vi "Write TCPClient.vi"(8 "error in (no error)":errorcluster, 10 "TCPClient.lvclass":refnum<class "TCPClient.lvclass">, 11 "MonoClient in":refnum<class "MonoClientCommunicator.lvclass">) -> (0 "error out":errorcluster, 3 "MonoClient out":refnum<class "MonoClientCommunicator.lvclass">)   [LabVIEW 2016, in "MonoClientCommunicator.lvclass"]
uses:
  MonoClientCommunicator.lvclass
  ts_labview_tcp/TCPClient/TCPClient.lvclass
  MonoClientCommunicator.lvclass/MonoClientCommunicator.ctl
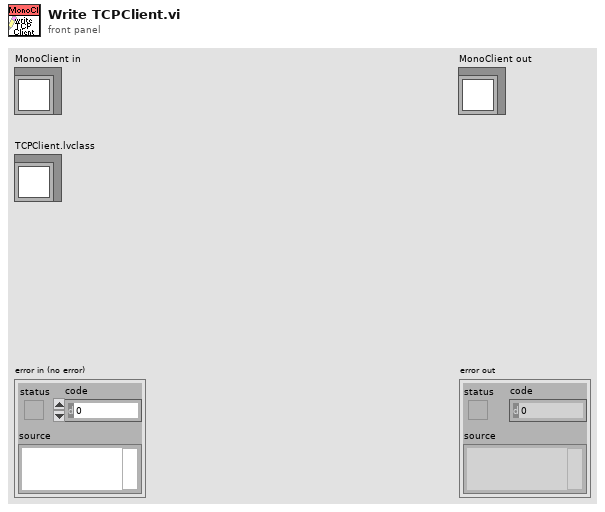
[diagram p1: front panel]
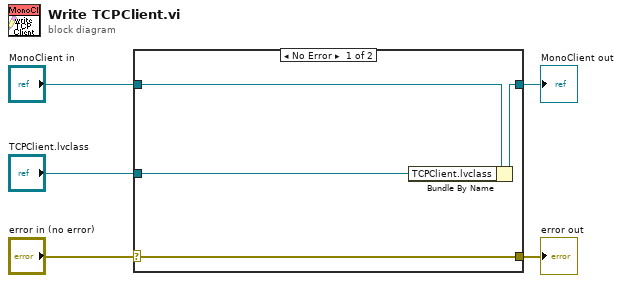
[diagram p0: block diagram]
diagram:
  n1 = case shown="No Error" "error in (no error)" {
    selector: "error in (no error)" -> [w9 w10]
    tunnel: [w9 w10] -> w4
    tunnel: [w7 w11] -> w2
    tunnel: "MonoClient in" -> [w8 w11]
    tunnel: "TCPClient.lvclass" -> [w6 _]
    frame No Error {
      n2 = Bundle By Name(cluster=w8, "TCPClient.lvclass"=w6) -> (w7:refnum<class "MonoClientCommunicator.lvclass">)
    }
    frame Error {
    }
  }
  "error out" <- w4
  "MonoClient out" <- w2
